vi "Initialize Buffer IDs.vi"(8 "error in":errorcluster, 10 "shared resources":refnum<class "Shared Resources.lvclass">, 11 "tx execution unit":refnum<class "Tx Execution Unit.lvclass">) -> (0 "error out":errorcluster, 3 "tx execution unit out":refnum<class "Tx Execution Unit.lvclass">)   [LabVIEW 2020, in "AIM MIL-STD-1553 Engine.lvlib" / "Implementation.lvlib" / "Tx Execution Unit.lvclass"]
uses:
  Tx Execution Unit.lvclass
  Tx Execution Unit.lvclass/Tx Execution Unit.ctl
  Shared Resources/Shared Resources.lvclass
  Shared/Direction.ctl
  <vilib>/NI VeriStand/Custom Device Tools/Custom Device Utility Library/Custom Device Utility Library.lvlib
  Interfaces/Shared Resources/Shared Resources.lvclass
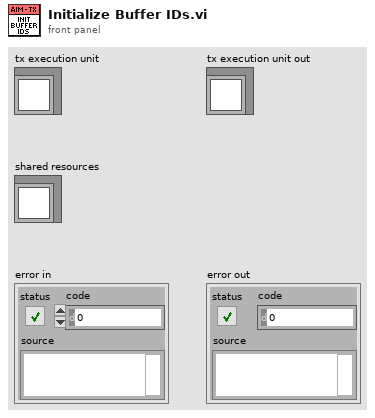
[diagram p1: front panel]
types:
  T1 = enum16{"unknown", "BC Message Buffer", "RT Message Buffer"}
  T2 = typedef "Direction.ctl" = enum16{"Rx", "Tx"}
  T3 = typedef "AIM MIL-STD-1553 Engine.lvlib/Implementation.lvlib/Shared Resources.lvclass/BC Subaddress to Buffer ID Map.ctl" = map{cluster{"TX Address":u8, "TX Subaddress":u8, "RX Address":u8, "RX Subaddress":u8}, cluster{"Buffer ID":u16}}
  T4 = typedef "AIM MIL-STD-1553 Engine.lvlib/Implementation.lvlib/Shared Resources.lvclass/RT Subaddress to Buffer ID Map.ctl" = map{cluster{"RT Address":u8, "Subaddress":u8, "Direction":T2}, cluster{"Buffer ID":u16}}
  T5 = typedef "AIM MIL-STD-1553 Engine.lvlib/Custom Device.lvlib/Compiled Message.ctl" = cluster{"Message Section Handle":T6, "First Parameter Index":i32, "Parameter Channel Handles":T6[], "Direction":T2, "Parameters":T7[], "Receiving RT Address":u8, "Receiving RT Sub-address":u8, "Transmitting RT Address":u8, "Transmitting RT Sub-address":u8, "Word Count":u8, "Buffer Type":enum16{"unknown", "BC Message Buffer", "RT Message Buffer"}, "Buffer ID":u16, "Terminal Type":enum16{"Bus Controller", "Remote Terminal"}, "Timestamp Enabled":bool, "Timestamp Channel Handle":T6}
  T6 = typedef "Custom Device API.lvlib/Custom Device Item Ref.ctl" = u64
  T7 = typedef "Parameter Definition.ctl" = cluster{"start index":i32, "size (bits)":i32, "encoding":enum16{"BNR", "BCD", "Discrete"}, "signed":bool, "multiplier":dbl, "offset":dbl}
  T8 = cluster{"Transmitting RT Address":u8, "Transmitting RT Sub-address":u8, "Direction":T2}
  T9 = cluster{"Transmitting RT Address":u8, "Transmitting RT Sub-address":u8, "Receiving RT Address":u8, "Receiving RT Sub-address":u8}
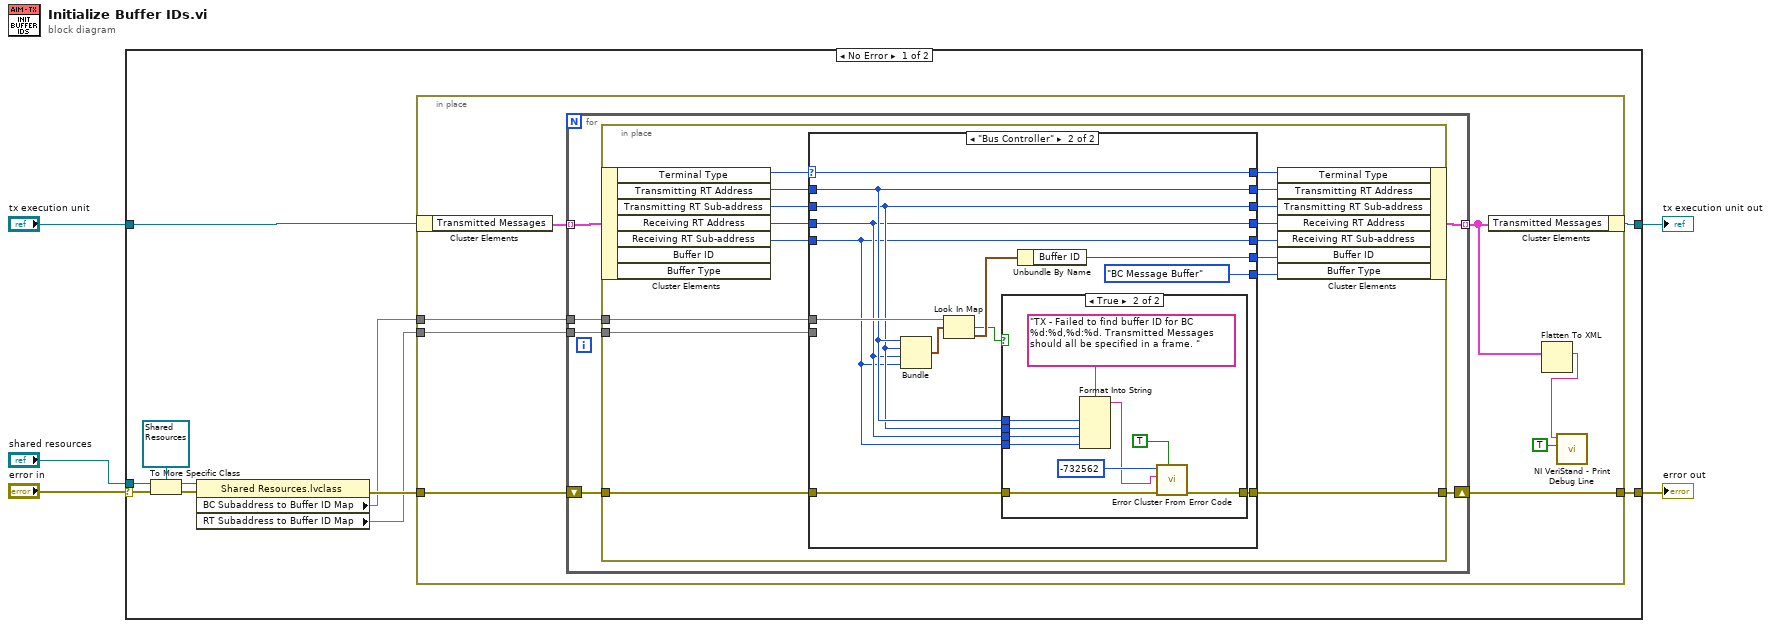
[diagram p0: block diagram]
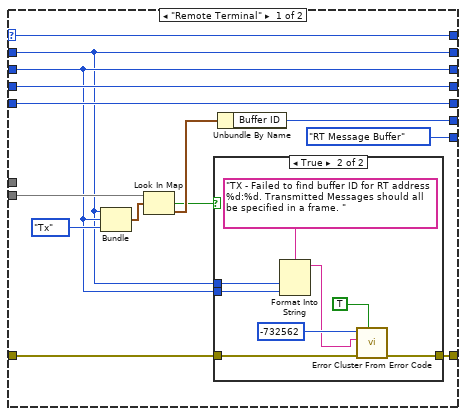
[diagram p2: hidden frame]
diagram:
  n1 = case shown="No Error" "error in" {
    selector: "error in" -> [w15 w94]
    tunnel: [w14 w95] -> w4
    tunnel: "shared resources" -> [w12 _]
    tunnel: "tx execution unit" -> [w10 w95]
    tunnel: [w8 w94] -> w1
    frame No Error {
      n2 = To More Specific Class(target class=refnum<class "Shared Resources.lvclass"> refnum ("specific class reference"), reference=w12, error in=w15) -> (specific class reference=w13:refnum<class "Shared Resources.lvclass">, error out=w16:errorcluster)
      n3 = property class="Shared Resources.lvclass"(reference=w13, error in=w16) -> (error out=w9:errorcluster, "BC Subaddress to Buffer ID Map"=w6:T3, "RT Subaddress to Buffer ID Map"=w7:T4)  [unwired: 1 out]
      n4 = in-place {
        in-place-border: w7 -> [w23]
        in-place-border: w9 -> [w22]
        in-place-border: [w21] -> w8
        in-place-border: w6 -> [w20]
        n5 = in-place-cluster #1(w10) -> ("Transmitted Messages"=w24:T5[])
        n6 = for {
          tunnel: w24 -> [w30] mode=indexing
          tunnel: [w29] -> w19 mode=indexing
          tunnel: w23 -> [w28]
          shift-right: [w26] -> w21
          shift-left: w22 -> [w27]
          tunnel: w20 -> [w25]
          n7 = in-place {
            in-place-border: w28 -> [w46]
            in-place-border: w27 -> [w45]
            in-place-border: [w44] -> w26
            in-place-border: w25 -> [w36]
            n8 = in-place-cluster #2(w30) -> ("Terminal Type"=w42:enum16{"Bus Controller", "Remote Terminal"}, "Transmitting RT Address"=w41:u8, "Transmitting RT Sub-address"=w40:u8, "Receiving RT Address"=w39:u8, "Receiving RT Sub-address"=w38:u8)  [unwired: 2 out]
            n9 = case shown="\"Bus Controller\"" w42 {
              selector: w42 -> [w52 w76]
              tunnel: w46 -> [w59 _]
              tunnel: [w56 w80] -> w31
              tunnel: w45 -> [w54 w78]
              tunnel: [w53 w77] -> w44
              tunnel: [w52 w76] -> w43
              tunnel: w41 -> [w47 w73]
              tunnel: w40 -> [w48 w72]
              tunnel: w39 -> [w50 w71]
              tunnel: w38 -> [w49 w70]
              tunnel: [T1."RT Message Buffer" ("Buffer Type") T1."BC Message Buffer" ("Buffer Type")] -> w37
              tunnel: [w50 w71] -> w33
              tunnel: [w49 w70] -> w32
              tunnel: [w48 w72] -> w34
              tunnel: [w47 w73] -> w35
              tunnel: w36 -> [_ w74]
              frame "Remote Terminal" {
                n10 = Bundle("Transmitting RT Address"=w47, "Transmitting RT Sub-address"=w48, "Direction"=Direction."Tx") -> (w60:T8)  [unwired: 1 in]
                n11 = Look In Map(map=w59, key=w60) -> (key not found?=w55:bool, value=w58:cluster{"Buffer ID":u16})  [unwired: 1 in]
                n12 = case shown="True" w55 {
                  tunnel: w47 -> [_ w68]
                  tunnel: w48 -> [_ w67]
                  tunnel: w54 -> [w61 w66]
                  tunnel: [w61 w65] -> w53
                  frame False {
                  }
                  frame True {
                    n13 = Format Into String(format string="TX - Failed to find buffer ID for RT address %d:%d. Transmitted Messages should all be specified in a frame. ", w68, w67) -> (resulting string=w63:string)  [unwired: 2 in, 1 out]
                    n14 = call <vilib>:"Error Cluster From Error Code.vi"("show call chain? (False)"=TRUE, "error in (no error)"=w66, "error message (\"\")"=w63, "error code (0)"=-732562) -> ("error out"=w65:errorcluster)  [unwired: 5 in]
                  }
                }
                n15 = Unbundle By Name(w58) -> ("Buffer ID"=w56:u16)
              }
              frame "Bus Controller" {
                n16 = Bundle("Transmitting RT Address"=w73, "Transmitting RT Sub-address"=w72, "Receiving RT Address"=w71, "Receiving RT Sub-address"=w70) -> (w82:T9)  [unwired: 1 in]
                n17 = Look In Map(map=w74, key=w82) -> (key not found?=w79:bool, value=w81:cluster{"Buffer ID":u16})  [unwired: 1 in]
                n18 = case shown="True" w79 {
                  tunnel: w73 -> [_ w92]
                  tunnel: w72 -> [_ w91]
                  tunnel: w78 -> [w83 w90]
                  tunnel: [w83 w89] -> w77
                  tunnel: w71 -> [_ w85]
                  tunnel: w70 -> [_ w84]
                  frame False {
                  }
                  frame True {
                    n19 = Format Into String(format string="TX - Failed to find buffer ID for BC %d:%d,%d:%d. Transmitted Messages should all be specified in a frame. ", w92, w91, w85, w84) -> (resulting string=w87:string)  [unwired: 2 in, 1 out]
                    n20 = call <vilib>:"Error Cluster From Error Code.vi"("show call chain? (False)"=TRUE, "error in (no error)"=w90, "error message (\"\")"=w87, "error code (0)"=-732562) -> ("error out"=w89:errorcluster)  [unwired: 5 in]
                  }
                }
                n21 = Unbundle By Name(w81) -> ("Buffer ID"=w80:u16)
              }
            }
            n22 = in-place-cluster #2("Terminal Type"=w43, "Transmitting RT Address"=w35, "Transmitting RT Sub-address"=w34, "Receiving RT Address"=w33, "Receiving RT Sub-address"=w32, "Buffer ID"=w31, "Buffer Type"=w37) -> (w29:T5)
          }
        }
        n23 = in-place-cluster #1("Transmitted Messages"=w19) -> (w14:refnum<class "Tx Execution Unit.lvclass">)
        n24 = Flatten To XML(6:w19) -> (2:w18:string)
        n25 = call <vilib>:"NI VeriStand - Print Debug Line.vi"("Add to log file? (F)"=TRUE, "Message"=w18) -> ()  [unwired: 9 in, 1 out]
      }
    }
    frame Error {
    }
  }
  "error out" <- w1
  "tx execution unit out" <- w4
